vi "calibration sub_VI.vi"(0 "VISA resource ESP32(COM4)":refnum<visa-resource-name>, 1 "Auto \ncalibration \nmode":bool, 2 "OUTPUT_F\nmode":bool, 3 "INPUT_F\nmode":bool, 5 "VISA resource \n2000(COM9)":refnum<visa-resource-name>="COM7", 11 "ESP32 error in":errorcluster, 12 "Calibration \nChannel":string, 13 "Ouput calibration\nparameter":string, 14 "Input calibration\nparameter":string) -> (4 "VISA resource ESP32(COM4) 2":refnum<visa-resource-name>, 6 "Calibration TX":string, 15 "error out":errorcluster)   [LabVIEW 2020]
uses:
  <instrlib>/Keithley 2600 Series/Public/Channel.ctl
  <instrlib>/Keithley 2000/Public/Configure/Configure DC Volts.vi
  <instrlib>/Keithley 2000/Keithley 2000.lvlib
  <instrlib>/Keithley 2600 Series/Keithley 2600 Series.lvlib
panel:
  in  "VISA resource \n2604B(COM10)":refnum<visa-resource-name>="COM7"
  out "OUTPUT or INPUT":u8(slide) scale=0.0..100.0
  out "CALIBRATION":u8(slide) scale=0.0..100.0
  in  "Channel (Channel A)":T1
  out "output parameter":dbl[](array[numeric]) format="%#.2f"
  out "Ouput 2600 read\n(each value)":dbl[][](array[numeric])
  out "Array 3":bool[](array[boolean])
  out "Array 2":i32[](array[numeric])
  in  "Ring":u16(ring)=1 items=["Channel 1"=1, "Channel 2"=2, "Channel 3"=3, "Channel 4"=4]
  # "CHANNEL"
  # "Calibration 吝"
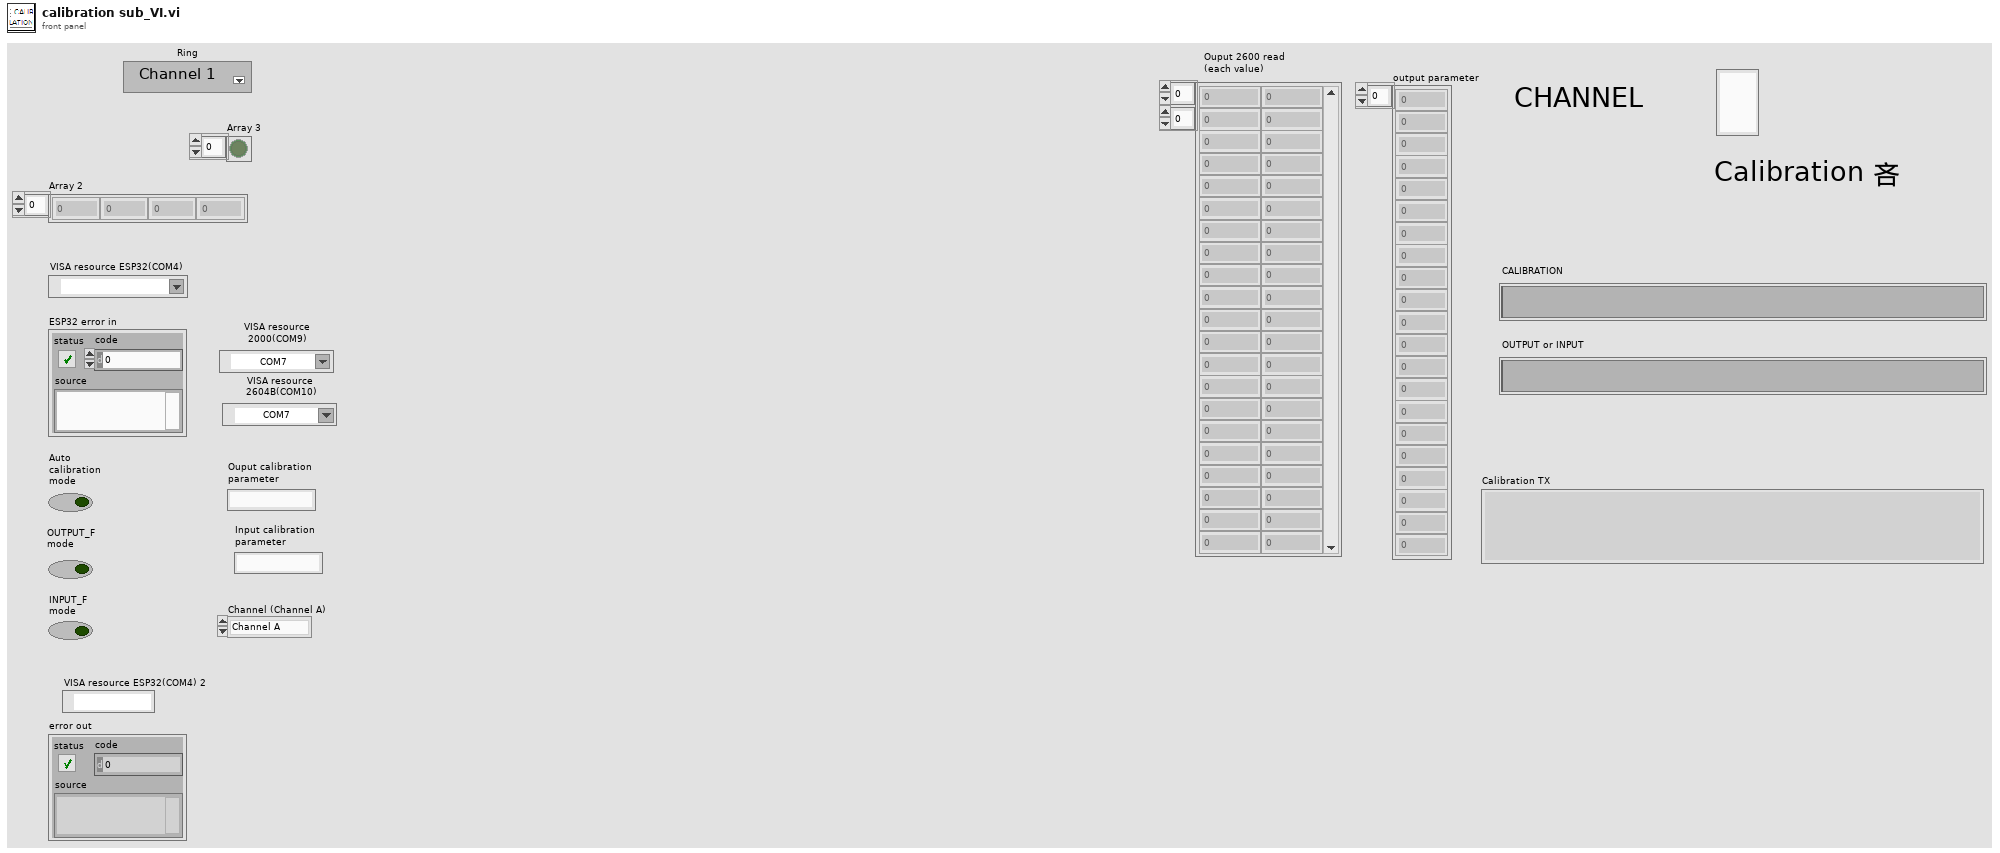
[diagram p1: front panel]
types:
  T1 = typedef "Keithley 2600 Series.lvlib/Channel.ctl" = enum32{"Channel A", "Channel B"}
  T2 = cluster{"Baud Rate":u32, "Parity":u16, "Data Bits":u16, "Stop Bits":u16, "Flow Control":u16}
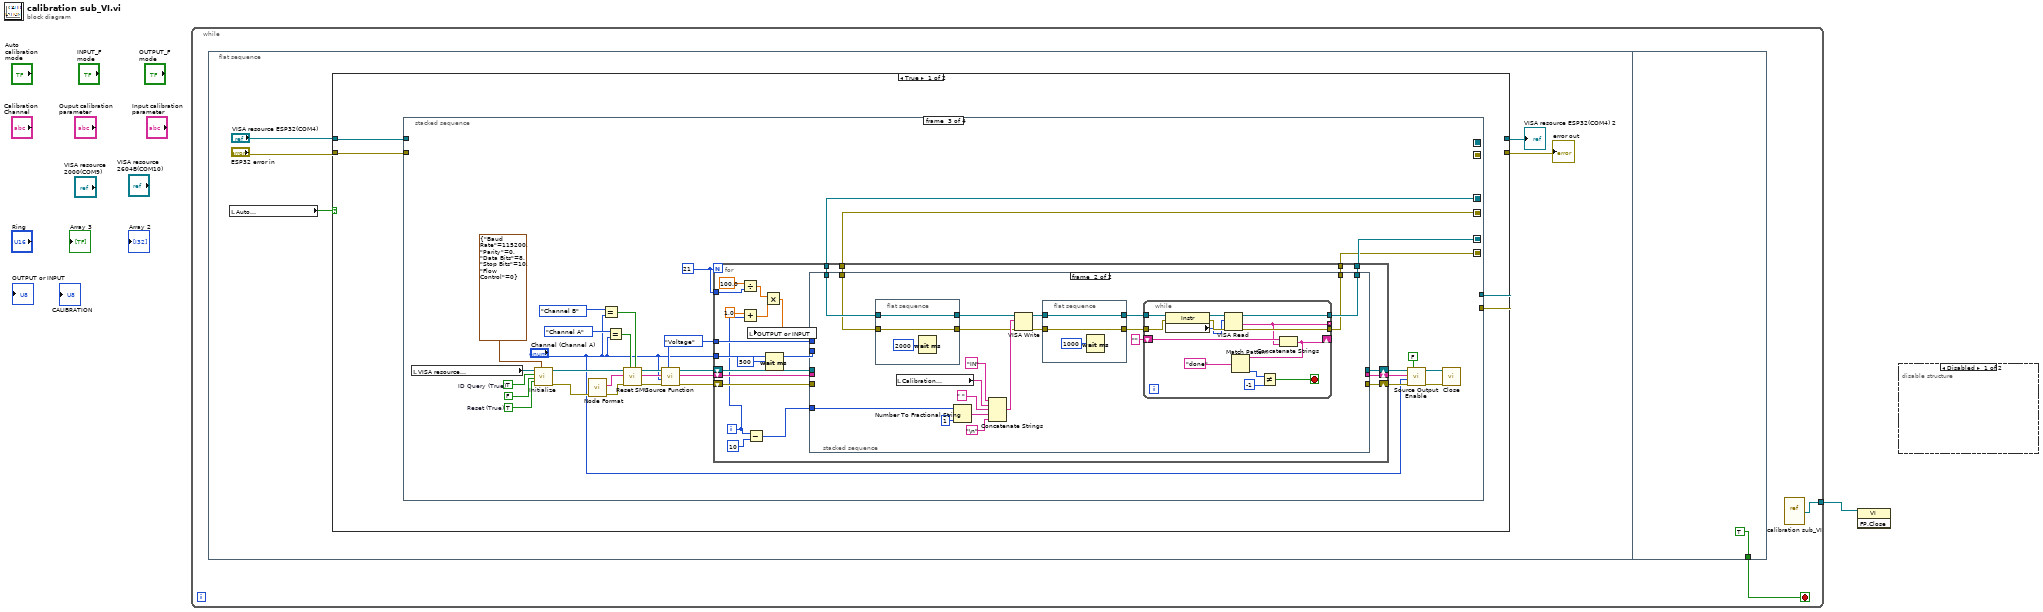
[diagram p0: block diagram]
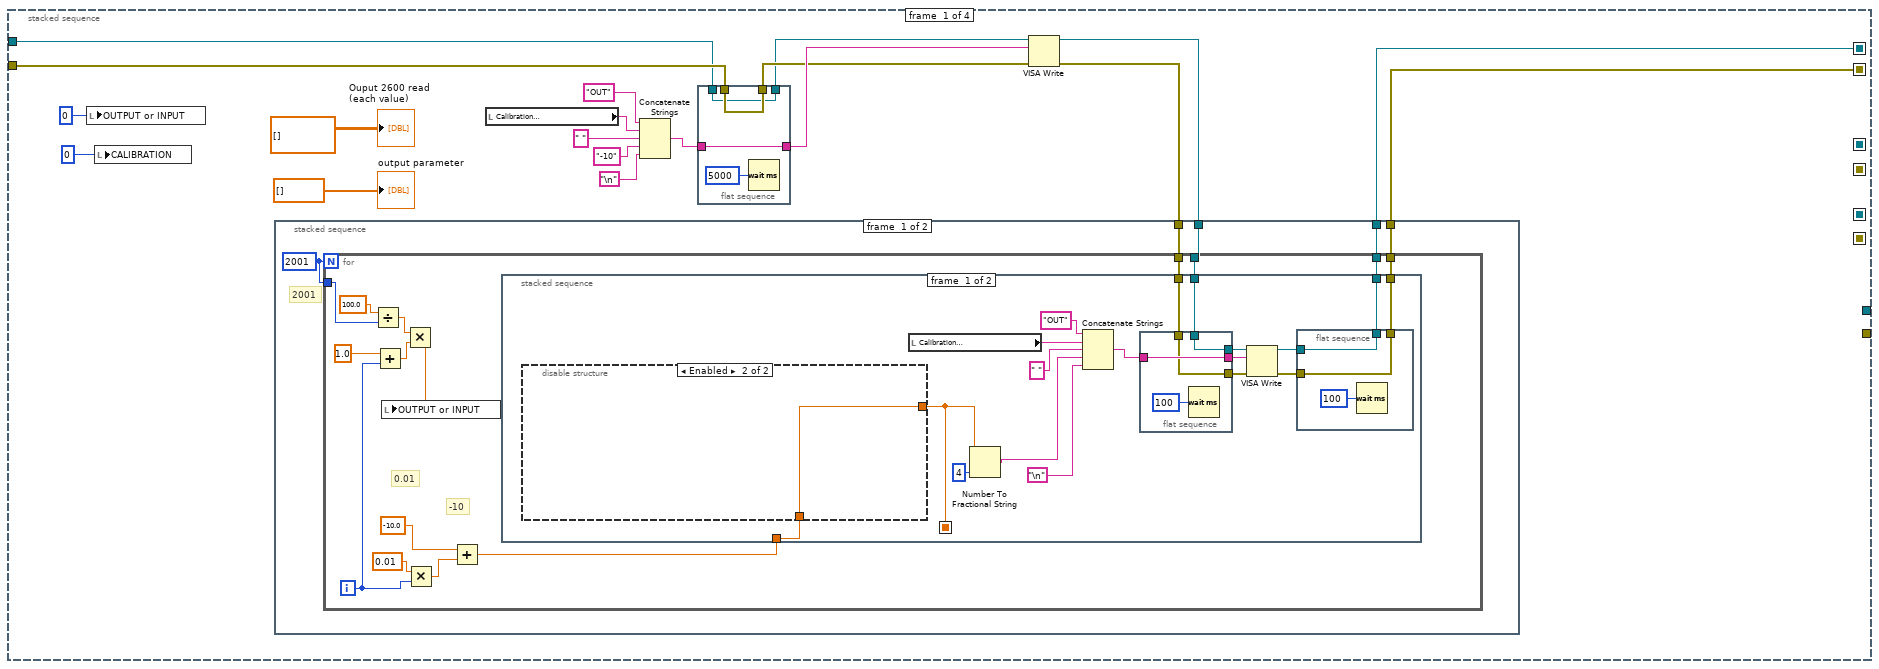
[diagram p3: hidden frame]
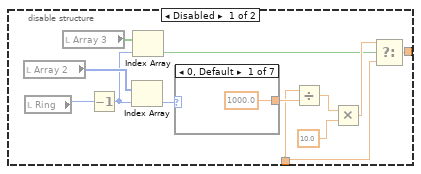
[diagram p4: hidden frame]
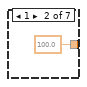
[diagram p5: hidden frame]
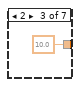
[diagram p6: hidden frame]
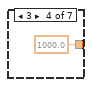
[diagram p7: hidden frame]
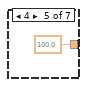
[diagram p8: hidden frame]
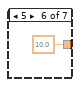
[diagram p9: hidden frame]
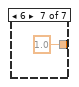
[diagram p10: hidden frame]
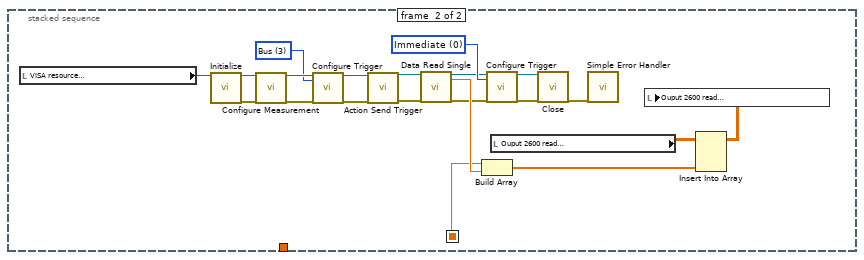
[diagram p11: hidden frame]
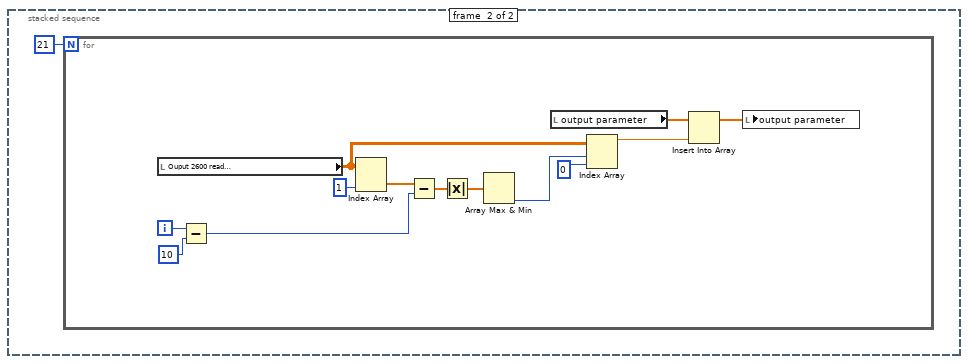
[diagram p12: hidden frame]
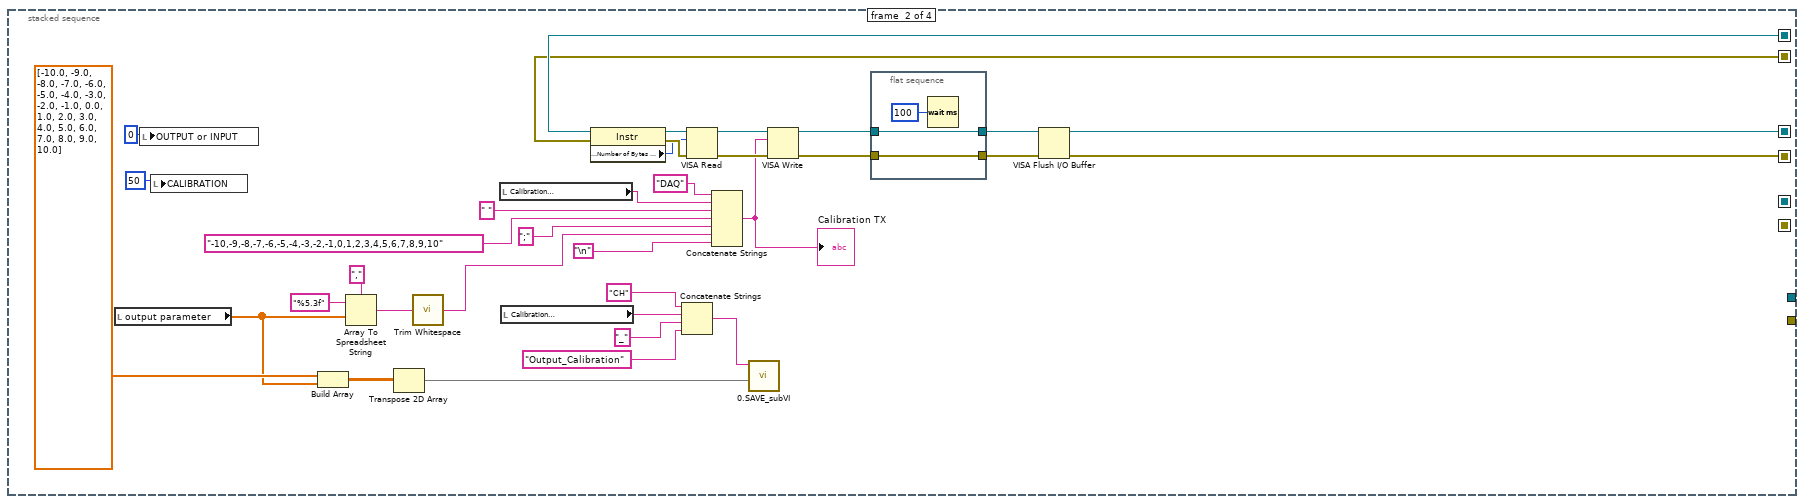
[diagram p13: hidden frame]
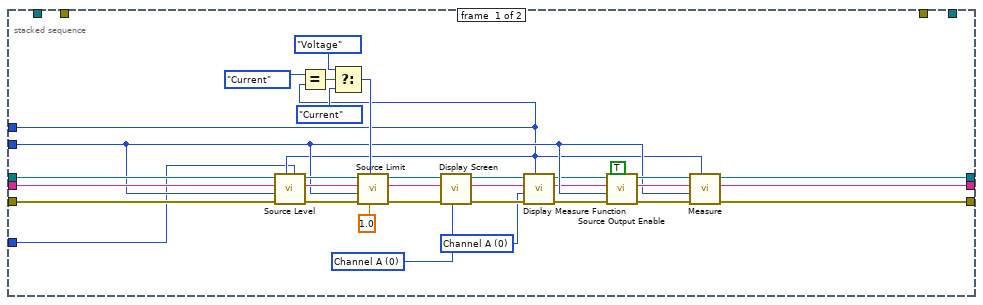
[diagram p14: hidden frame]
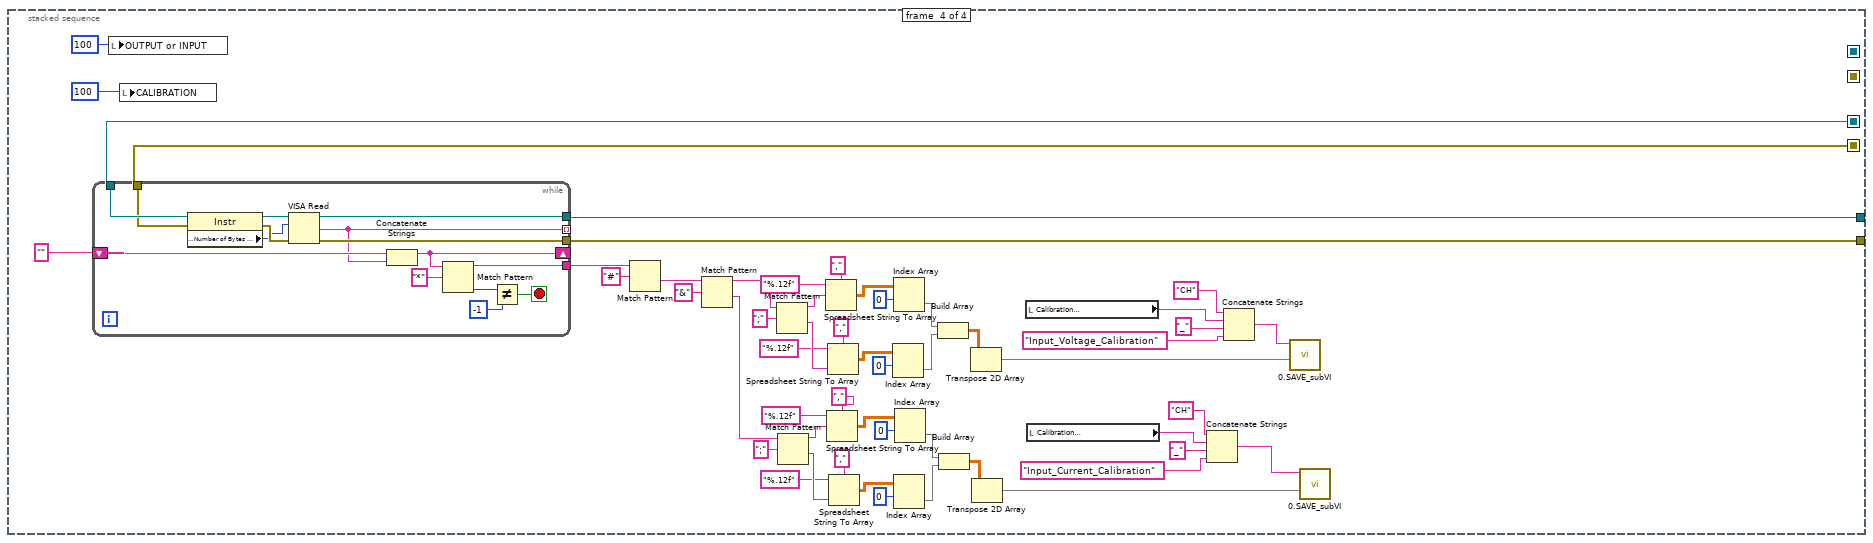
[diagram p15: hidden frame]
diagram:
  n1 = while {
    tunnel: [w2] -> w1
    stop <- w3 stop-if-true
    n2 = flat-sequence {
      tunnel: [TRUE] -> w3
      frame #0 {
        n3 = local read "Auto \ncalibration \nmode"() -> (w4:bool)
        n4 = case shown="True" w4 {
          tunnel: "VISA resource ESP32(COM4)" -> [w12 w369]
          tunnel: [w10 w369] -> w6
          tunnel: [w9 w368] -> w5
          tunnel: "ESP32 error in" -> [w11 w368]
          frame True {
            n5 = stacked-sequence {
              seq-local: [w30 _ _ _] -> [_ w161 _ _]
              seq-local: [w29 _ _ _] -> [_ w160 _ _]
              seq-local: [_ w164 _ _] -> [_ _ w179 _]
              seq-local: [_ w165 _ _] -> [_ _ w180 _]
              seq-local: [_ _ w178 _] -> [_ _ _ w351]
              seq-local: [_ _ w177 _] -> [_ _ _ w350]
              tunnel: w12 -> [w21 _ _ _]
              tunnel: w11 -> [w22 _ _ _]
              tunnel: [_ _ _ w339] -> w10
              tunnel: [_ _ _ w338] -> w9
              frame #0 {
                n6 = local write "OUTPUT or INPUT"(u8 0 ("Slide 2")) -> ()
                n7 = local write "CALIBRATION"(u8 0 ("Slide")) -> ()
                n8 = local read "Calibration \nChannel"() -> (w18:string)
                n9 = Concatenate Strings("OUT" ("string"), w18, " " ("string"), "-10" ("string"), "\n") -> (w25:string)
                n10 = flat-sequence {
                  tunnel: w25 -> [w34]
                  tunnel: [w34] -> w24
                  tunnel: [w33] -> w23
                  tunnel: w22 -> [w33]
                  tunnel: w21 -> [w32]
                  tunnel: [w32] -> w20
                  frame #0 {
                    n11 = Wait (ms)(milliseconds to wait=u32 5000) -> ()  [unwired: 1 out]
                  }
                }
                n12 = VISA Write(VISA resource name=w20, write buffer=w24, error in (no error)=w23) -> (VISA resource name out=w27:refnum<visa-resource-name>, error out=w26:errorcluster)  [unwired: 1 out]
                n13 = stacked-sequence {
                  tunnel: w27 -> [w40 _]
                  tunnel: w26 -> [w39 _]
                  tunnel: [w38 _] -> w30
                  tunnel: [w37 _] -> w29
                  frame #0 {
                    w36 = 2001
                    # "2001"
                    n14 = for {
                      N: w36 -> [_]
                      tunnel: w40 -> [w55]
                      tunnel: w39 -> [w54]
                      tunnel: [w53] -> w38
                      tunnel: [w52] -> w37
                      tunnel: w36 -> [w46]
                      i -> [w44]
                      # "-10"
                      # "0.01"
                      n15 = Divide(x=100.0, y=w46) -> (x/y=w42:dbl)
                      n16 = Add(x=1.0, y=w44) -> (x+y=w43:dbl)
                      n17 = Multiply(x=w42, y=w43) -> (x*y=w41:dbl)
                      n18 = local write "OUTPUT or INPUT"(w41) -> ()
                      n19 = Multiply(x=0.01, y=w44) -> (x*y=w49:dbl)
                      n20 = Add(x=-10.0, y=w49) -> (x+y=w48:dbl)
                      n21 = stacked-sequence {
                        seq-local: [w69 _] -> [_ w107]
                        tunnel: w48 -> [w70 _]
                        tunnel: w55 -> [w65 _]
                        tunnel: w54 -> [w63 _]
                        tunnel: [w62 _] -> w53
                        tunnel: [w60 _] -> w52
                        frame #0 {
                          n22 = disable-structure shown="Enabled" {
                            disable-tunnel: w70 -> [w75 w93]
                            disable-tunnel: [w74 w93] -> w69
                            frame Disabled {
                              n23 = local read "Array 2"() -> (w82:i32[])
                              n24 = local read "Ring"() -> (w83:u16)
                              n25 = local read "Array 3"() -> (w79:bool[])
                              n26 = Decrement(x=w83) -> (x-1=w77:u16)
                              n27 = Index Array(array=w82, index=w77) -> (element=w81:i32)
                              n28 = Index Array(array=w79, index=w77) -> (element=w78:bool)
                              n29 = case shown="0, Default" w81 {
                                tunnel: [1000.0 100.0 10.0 1000.0 100.0 10.0 1.0] -> w84
                                frame 0, Default {
                                }
                                frame 1 {
                                }
                                frame 2 {
                                }
                                frame 3 {
                                }
                                frame 4 {
                                }
                                frame 5 {
                                }
                                frame 6 {
                                }
                              }
                              n30 = Divide(x=w75, y=w84) -> (x/y=w85:dbl)
                              n31 = Multiply(x=w85, y=10.0) -> (x*y=w80:dbl)
                              n32 = Select(t=w80, s=w78, f=w75) -> (s? t:f=w74:dbl)
                            }
                            frame Enabled {
                            }
                          }
                          n33 = local read "Calibration \nChannel"() -> (w57:string)
                          n34 = Number To Fractional String(number=w69, precision (6)=i16 4) -> (F-format string=w73:string)  [unwired: 2 in]
                          n35 = Concatenate Strings("OUT" ("string"), w57, " " ("string"), w73, "\n") -> (w67:string)
                          n36 = flat-sequence {
                            tunnel: [w99] -> w68
                            tunnel: w67 -> [w99]
                            tunnel: [w98] -> w66
                            tunnel: w65 -> [w98]
                            tunnel: [w97] -> w64
                            tunnel: w63 -> [w97]
                            frame #0 {
                              n37 = Wait (ms)(milliseconds to wait=u32 100) -> ()  [unwired: 1 out]
                            }
                          }
                          n38 = VISA Write(VISA resource name=w66, write buffer=w68, error in (no error)=w64) -> (VISA resource name out=w61:refnum<visa-resource-name>, error out=w59:errorcluster)  [unwired: 1 out]
                          n39 = flat-sequence {
                            tunnel: [w95] -> w62
                            tunnel: w61 -> [w95]
                            tunnel: [w94] -> w60
                            tunnel: w59 -> [w94]
                            frame #0 {
                              n40 = Wait (ms)(milliseconds to wait=u32 100) -> ()  [unwired: 1 out]
                            }
                          }
                        }
                        frame #1 {
                          w106 = u16 0 items=["Immediate", "Timer", "Manual", "Bus", "External"] ("Source (0: Immediate)")
                          w116 = u16 3 items=["Immediate", "Timer", "Manual", "Bus", "External"] ("Source (0: Immediate)")
                          n41 = local read "VISA resource \n2000(COM9)"() -> (w101:refnum<visa-resource-name>)
                          n42 = call <instrlib>:"Initialize.vi"("VISA resource name"=w101) -> ("VISA resource name out"=w120:refnum<visa-resource-name>, "error out"=w121:errorcluster)  [unwired: 17 in]
                          n43 = call-poly <instrlib>:"Configure Measurement.vi"("VISA resource name"=w120, "error in (no error)"=w121) -> ("VISA resource name out"=w117:refnum<visa-resource-name>, "error out"=w118:errorcluster)  [unwired: 16 in]
                          n44 = call <instrlib>:"Configure Trigger.vi"("VISA resource name"=w117, "Source (0: Immediate)"=w116, "error in (no error)"=w118) -> ("VISA resource name out"=w115:refnum<visa-resource-name>, "error out"=w114:errorcluster)  [unwired: 15 in]
                          n45 = call <instrlib>:"Action Send Trigger.vi"("VISA resource name"=w115, "error in (no error)"=w114) -> ("VISA resource name out"=w112:refnum<visa-resource-name>, "error out"=w113:errorcluster)  [unwired: 16 in]
                          n46 = call <instrlib>:"Data Read Single.vi"("VISA resource name"=w112, "error in (no error)"=w113) -> ("VISA resource name out"=w102:refnum<visa-resource-name>, "Measurement"=w109:dbl, "error out"=w103:errorcluster)  [unwired: 13 in, 2 out]
                          n47 = Build Array(w107, w109) -> (w108:dbl[])
                          n48 = call <instrlib>:"Configure Trigger.vi"("VISA resource name"=w102, "Source (0: Immediate)"=w106, "error in (no error)"=w103) -> ("VISA resource name out"=w105:refnum<visa-resource-name>, "error out"=w104:errorcluster)  [unwired: 15 in]
                          n49 = local read "Ouput 2600 read\n(each value)"() -> (w110:dbl[][])
                          n50 = call <instrlib>:"Close.vi"("VISA resource name"=w105, "error in (no error)"=w104) -> ("error out"=w119:errorcluster)  [unwired: 17 in]
                          n51 = call <vilib>:"Simple Error Handler.vi"("error in (no error)"=w119) -> ()  [unwired: 4 in, 5 out]
                          n52 = Insert Into Array(array=w110, new element=w108) -> (w111:dbl[][])  [unwired: 2 in]
                          n53 = local write "Ouput 2600 read\n(each value)"(w111) -> ()
                        }
                      }
                    }
                  }
                  frame #1 {
                    n54 = for {
                      N: 21 -> [_]
                      i -> [w135]
                      n55 = local read "Ouput 2600 read\n(each value)"() -> (w123:dbl[][])
                      n56 = Subtract(x=w135, y=10) -> (x-y=w131:i32)
                      n57 = Index Array(array=w123, index (col)=1 ("disabled index (col)")) -> (element=w132:dbl[])  [unwired: 1 in]
                      n58 = Subtract(x=w132, y=w131) -> (x-y=w130:dbl[])
                      n59 = Absolute Value(x=w130) -> (abs(x)=w129:dbl[])
                      n60 = Array Max & Min(array=w129) -> (min index (indices)=w124:i32)  [unwired: 3 out]
                      n61 = local read "output parameter"() -> (w127:dbl[])
                      n62 = Index Array(array=w123, index (row)=w124, index (col)=0 ("disabled index (col)")) -> (element=w126:dbl)
                      n63 = Insert Into Array(array=w127, new element=w126) -> (w128:dbl[])  [unwired: 1 in]
                      n64 = local write "output parameter"(w128) -> ()
                    }
                  }
                }
                "output parameter" <- dbl[] [] ("array")
                "Ouput 2600 read\n(each value)" <- dbl[][] [] ("array")
              }
              frame #1 {
                n65 = local read "output parameter"() -> (w166:dbl[])
                n66 = local write "OUTPUT or INPUT"(u8 0 ("Slide 2")) -> ()
                n67 = local write "CALIBRATION"(u8 50 ("Slide")) -> ()
                n68 = Build Array(dbl[] [-10.0, -9.0, -8.0, -7.0, -6.0, -5.0, -4.0, -3.0, -2.0, -1.0, 0.0, 1.0, 2.0, 3.0, 4.0, 5.0, 6.0, 7.0, 8.0, 9.0, 10.0], w166) -> (w168:dbl[][])
                n69 = Array To Spreadsheet String(delimiter (Tab)=",", array=w166, 3:"%5.3f" ("format string")) -> (spreadsheet string=w163:string)
                n70 = Transpose 2D Array(2D array=w168) -> (transposed array=w151:dbl[][])
                n71 = call <vilib>:"Trim Whitespace.vi"("string"=w163) -> ("trimmed string"=w148:string)  [unwired: 1 in]
                n72 = local read "Calibration \nChannel"() -> (w142:string)
                n73 = local read "Calibration \nChannel"() -> (w139:string)
                n74 = property class="Instr"(reference=w161, error in=w160) -> (reference out=w159:refnum<visa-resource-name>, error out=w158:errorcluster, "Serial Settings:Number of Bytes at Serial Port"=w157:u32)
                n75 = Concatenate Strings("CH" ("time format string (%c)"), w139, "_" ("time format string (%c)"), "Output_Calibration" ("time format string (%c)")) -> (w144:string)
                n76 = VISA Read(VISA resource name=w159, byte count=w157, error in (no error)=w158) -> (VISA resource name out=w156:refnum<visa-resource-name>, error out=w155:errorcluster)  [unwired: 2 out]
                n77 = Concatenate Strings("DAQ" ("string"), w142, " " ("string"), "-10,-9,-8,-7,-6,-5,-4,-3,-2,-1,0,1,2,3,4,5,6,7,8,9,10" ("string"), ";" ("string"), w148, "\n") -> (w146:string)
                "Calibration TX" <- w146
                n78 = call "0.SAVE_subVI.vi"("2D data"=w151, "file name"=w144) -> ()  [unwired: 10 in]
                n79 = VISA Write(VISA resource name=w156, write buffer=w146, error in (no error)=w155) -> (VISA resource name out=w152:refnum<visa-resource-name>, error out=w154:errorcluster)  [unwired: 1 out]
                n80 = flat-sequence {
                  tunnel: [w173] -> w162
                  tunnel: w154 -> [w173]
                  tunnel: [w172] -> w153
                  tunnel: w152 -> [w172]
                  frame #0 {
                    n81 = Wait (ms)(milliseconds to wait=u32 100) -> ()  [unwired: 1 out]
                  }
                }
                n82 = VISA Flush I/O Buffer(VISA resource name=w153, error in (no error)=w162) -> (VISA resource name out=w165:refnum<visa-resource-name>, error out=w164:errorcluster)  [unwired: 1 in]
              }
              frame #2 {
                w175 = 21
                w188 = enum32{"Current", "Voltage"}."Voltage" ("Source Function (Current)")
                w204 = TRUE  # Reset (True)
                w205 = TRUE  # ID Query (True)
                n83 = local read "VISA resource \n2604B(COM10)"() -> (w174:refnum<visa-resource-name>)
                n84 = call <instrlib>:"Initialize.vi"("Reset (True)"=w204, "Serial Configuration"=T2 {"Baud Rate"=115200, "Parity"=0, "Data Bits"=8, "Stop Bits"=10, "Flow Control"=0}, "Error Query (False)"=FALSE, "ID Query (True)"=w205, "VISA resource name"=w174) -> ("error out"=w193:errorcluster, "VISA resource name out"=w202:refnum<visa-resource-name>)  [unwired: 1 in, 4 out]
                n85 = call <instrlib>:"Node Format.vi"("error in"=w193) -> ("error out"=w192:errorcluster, "Formatted Node"=w194:string)  [unwired: 1 in, 8 out]
                n86 = Equal?(x=enum32{"Channel A", "Channel B"}."Channel B", y="Channel (Channel A)") -> (x = y?=w198:bool)
                n87 = Equal?(x=enum32{"Channel A", "Channel B"}."Channel A", y="Channel (Channel A)") -> (x = y?=w199:bool)
                n88 = call <instrlib>:"Reset SMU.vi"("SMU B (No)"=w198, "SMU A (No)"=w199, "error in (no error)"=w192, "Node In"=w194, "VISA resource name"=w202) -> ("error out"=w197:errorcluster, "Node Out"=w195:string, "VISA resource name out"=w196:refnum<visa-resource-name>)  [unwired: 4 out]
                n89 = call <instrlib>:"Source Function.vi"("Function (Current)"=w188, "error in (no error)"=w197, "Channel (Channel A)"="Channel (Channel A)", "Node In"=w195, "VISA resource name"=w196) -> ("error out"=w189:errorcluster, "Node Out"=w191:string, "VISA resource name out"=w190:refnum<visa-resource-name>)  [unwired: 4 out]
                n90 = for {
                  N: w175 -> [_]
                  tunnel: "Channel (Channel A)" -> [w221]
                  tunnel: w188 -> [w220]
                  shift-right: [w222] -> w183
                  shift-left: w191 -> [w227]
                  shift-right: [w224] -> w184
                  shift-left: w190 -> [w226]
                  shift-right: [w223] -> w182
                  shift-left: w189 -> [w225]
                  tunnel: [w217] -> w178
                  tunnel: [w216] -> w177
                  tunnel: w180 -> [w215]
                  tunnel: w179 -> [w214]
                  tunnel: w175 -> [w211]
                  i -> [w209]
                  n91 = Divide(x=100.0, y=w211) -> (x/y=w208:dbl)
                  n92 = Add(x=1.0, y=w209) -> (x+y=w207:dbl)
                  n93 = Subtract(x=w209, y=10) -> (x-y=w219:i32)
                  n94 = Multiply(x=w208, y=w207) -> (x*y=w206:dbl)
                  n95 = local write "OUTPUT or INPUT"(w206) -> ()
                  n96 = Wait (ms)(milliseconds to wait=u32 500) -> ()  [unwired: 1 out]
                  n97 = stacked-sequence {
                    tunnel: w227 -> [w260 _]
                    tunnel: w226 -> [w259 _]
                    tunnel: w225 -> [w258 _]
                    tunnel: [w253 _] -> w224
                    tunnel: [w252 _] -> w223
                    tunnel: [w248 _] -> w222
                    tunnel: w221 -> [w243 _]
                    tunnel: w220 -> [w230 _]
                    tunnel: w219 -> [w229 w276]
                    tunnel: [_ w279] -> w217
                    tunnel: [_ w278] -> w216
                    tunnel: w215 -> [_ w277]
                    tunnel: w214 -> [_ w275]
                    frame #0 {
                      w231 = u16 0 items=["Channel A", "Channel B"] ("Channel (Channel A)")
                      w241 = u16 0 items=["Channel A", "Channel B", "Channels A & B", "User"] ("Screen (Channels A & B)")
                      n98 = call <instrlib>:"Source Level.vi"("Level (0.000)"=w229, "Function (Current)"=w230, "error in (no error)"=w258, "Channel (Channel A)"=w243, "Node In"=w260, "VISA resource name"=w259) -> ("error out"=w257:errorcluster, "Node Out"=w250:string, "VISA resource name out"=w256:refnum<visa-resource-name>)  [unwired: 3 out]
                      n99 = Equal?(x=enum32{"Current", "Voltage"}."Current", y=w230) -> (x = y?=w246:bool)
                      n100 = Select(t=enum32{"Current", "Voltage"}."Voltage" ("x"), s=w246, f=enum32{"Current", "Voltage"}."Current") -> (s? t:f=w244:enum32{"Current", "Voltage"})
                      n101 = call <instrlib>:"Source Limit.vi"("Limit (0.000)"=1.0, "Function (Current)"=w244, "error in (no error)"=w257, "Channel (Channel A)"=w243, "Node In"=w250, "VISA resource name"=w256) -> ("error out"=w238:errorcluster, "Node Out"=w239:string, "VISA resource name out"=w240:refnum<visa-resource-name>)  [unwired: 3 out]
                      n102 = call <instrlib>:"Display Screen.vi"("Screen (Channels A & B)"=w241, "error in (no error)"=w238, "Node In"=w239, "VISA resource name"=w240) -> ("error out"=w235:errorcluster, "Node Out"=w236:string, "VISA resource name out"=w237:refnum<visa-resource-name>)  [unwired: 4 in, 1 out]
                      n103 = call <instrlib>:"Display Measure Function.vi"("Function (Current)"=w230, "error in (no error)"=w235, "Channel (Channel A)"=w231, "Node In"=w236, "VISA resource name"=w237) -> ("error out"=w232:errorcluster, "Node Out"=w233:string, "VISA resource name out"=w234:refnum<visa-resource-name>)  [unwired: 3 in, 1 out]
                      n104 = call <instrlib>:"Source Output Enable.vi"("Output (Off)"=TRUE, "error in (no error)"=w232, "Channel (Channel A)"=w243, "Node In"=w233, "VISA resource name"=w234) -> ("error out"=w255:errorcluster, "Node Out"=w249:string, "VISA resource name out"=w254:refnum<visa-resource-name>)  [unwired: 4 out]
                      n105 = call <instrlib>:"Measure.vi"("Function (Current)"=w230, "error in (no error)"=w255, "Channel (Channel A)"=w243, "Node In"=w249, "VISA resource name"=w254) -> ("error out"=w252:errorcluster, "Node Out"=w248:string, "VISA resource name out"=w253:refnum<visa-resource-name>)  [unwired: 2 in, 2 out]
                    }
                    frame #1 {
                      n106 = flat-sequence {
                        tunnel: [w299] -> w269
                        tunnel: w277 -> [w299]
                        tunnel: w275 -> [w297]
                        tunnel: [w297] -> w267
                        frame #0 {
                          n107 = Wait (ms)(milliseconds to wait=u32 2000) -> ()  [unwired: 1 out]
                        }
                      }
                      n108 = local read "Calibration \nChannel"() -> (w262:string)
                      n109 = Number To Fractional String(number=w276, precision (6)=i16 1) -> (F-format string=w271:string)  [unwired: 2 in]
                      n110 = Concatenate Strings("IN" ("string"), w262, " " ("string"), w271, "\n") -> (w268:string)
                      n111 = VISA Write(VISA resource name=w269, write buffer=w268, error in (no error)=w267) -> (VISA resource name out=w274:refnum<visa-resource-name>, error out=w273:errorcluster)  [unwired: 1 out]
                      n112 = flat-sequence {
                        tunnel: [w282] -> w266
                        tunnel: w274 -> [w282]
                        tunnel: w273 -> [w280]
                        tunnel: [w280] -> w265
                        frame #0 {
                          n113 = Wait (ms)(milliseconds to wait=u32 1000) -> ()  [unwired: 1 out]
                        }
                      }
                      n114 = while {
                        tunnel: [w296] -> w279
                        tunnel: w266 -> [w293]
                        tunnel: w265 -> [w292]
                        tunnel: [w291] -> w278
                        tunnel: [w284] -> _ mode=indexing
                        shift-right: [w283] -> _
                        shift-left: "" -> [w285]
                        stop <- w286 stop-if-true
                        n115 = property class="Instr"(reference=w293, error in=w292) -> (reference out=w295:refnum<visa-resource-name>, error out=w294:errorcluster, "Serial Settings:Number of Bytes at Serial Port"=w290:u32)
                        n116 = VISA Read(VISA resource name=w295, byte count=w290, error in (no error)=w294) -> (VISA resource name out=w296:refnum<visa-resource-name>, read buffer=w284:string, error out=w291:errorcluster)  [unwired: 1 out]
                        n117 = Concatenate Strings(w285, w284) -> (w283:string)
                        n118 = Match Pattern(string=w283, regular expression="done" ("x")) -> (offset past match=w288:i32)  [unwired: 1 in, 3 out]
                        n119 = Not Equal?(x=w288, y=-1) -> (x != y?=w286:bool)
                      }
                    }
                  }
                }
                n120 = call <instrlib>:"Source Output Enable.vi"("Output (Off)"=FALSE, "error in (no error)"=w182, "Channel (Channel A)"="Channel (Channel A)", "Node In"=w183, "VISA resource name"=w184) -> ("error out"=w186:errorcluster, "VISA resource name out"=w187:refnum<visa-resource-name>)  [unwired: 5 out]
                n121 = call <instrlib>:"Close.vi"("error in (no error)"=w186, "VISA resource name"=w187) -> ()  [unwired: 10 out]
              }
              frame #3 {
                n122 = while {
                  tunnel: [w367] -> w339
                  tunnel: [w364] -> w338
                  tunnel: [w358] -> _ mode=indexing
                  shift-right: [w357] -> _
                  shift-left: "" -> [w359]
                  tunnel: w351 -> [w355]
                  tunnel: w350 -> [w354]
                  tunnel: [w353] -> w334
                  stop <- w356 stop-if-true
                  n123 = property class="Instr"(reference=w355, error in=w354) -> (reference out=w366:refnum<visa-resource-name>, error out=w365:errorcluster, "Serial Settings:Number of Bytes at Serial Port"=w363:u32)
                  n124 = VISA Read(VISA resource name=w366, byte count=w363, error in (no error)=w365) -> (VISA resource name out=w367:refnum<visa-resource-name>, read buffer=w358:string, error out=w364:errorcluster)  [unwired: 1 out]
                  n125 = Concatenate Strings(w359, w358) -> (w357:string)
                  n126 = Match Pattern(string=w357, regular expression="*" ("x")) -> (before substring=w353:string, offset past match=w361:i32)  [unwired: 1 in, 2 out]
                  n127 = Not Equal?(x=w361, y=-1) -> (x != y?=w356:bool)
                }
                n128 = local write "OUTPUT or INPUT"(u8 100 ("Slide 2")) -> ()
                n129 = local write "CALIBRATION"(u8 100 ("Slide")) -> ()
                n130 = Match Pattern(string=w334, regular expression="#") -> (after substring=w336:string)  [unwired: 1 in, 3 out]
                n131 = Match Pattern(string=w336, regular expression="&") -> (before substring=w319:string, after substring=w304:string)  [unwired: 1 in, 2 out]
                n132 = Match Pattern(string=w319, regular expression=";") -> (before substring=w322:string, after substring=w325:string)  [unwired: 1 in, 2 out]
                n133 = Match Pattern(string=w304, regular expression=";") -> (before substring=w307:string, after substring=w310:string)  [unwired: 1 in, 2 out]
                n134 = Spreadsheet String To Array(delimiter (Tab)=",", format string="%.12f", spreadsheet string=w322) -> (array=w326:dbl[][])  [unwired: 1 in]
                n135 = Spreadsheet String To Array(delimiter (Tab)=",", format string="%.12f", spreadsheet string=w307) -> (array=w311:dbl[][])  [unwired: 1 in]
                n136 = Spreadsheet String To Array(delimiter (Tab)=",", format string="%.12f", spreadsheet string=w325) -> (array=w331:dbl[][])  [unwired: 1 in]
                n137 = Spreadsheet String To Array(delimiter (Tab)=",", format string="%.12f", spreadsheet string=w310) -> (array=w316:dbl[][])  [unwired: 1 in]
                n138 = Index Array(array=w331, index (row)=0 ("disabled index (col)")) -> (element=w332:dbl[])  [unwired: 1 in]
                n139 = Index Array(array=w326, index (row)=0 ("disabled index (col)")) -> (element=w327:dbl[])  [unwired: 1 in]
                n140 = Index Array(array=w316, index (row)=0 ("disabled index (col)")) -> (element=w317:dbl[])  [unwired: 1 in]
                n141 = Index Array(array=w311, index (row)=0 ("disabled index (col)")) -> (element=w312:dbl[])  [unwired: 1 in]
                n142 = Build Array(w327, w332) -> (w329:dbl[][])
                n143 = Build Array(w312, w317) -> (w314:dbl[][])
                n144 = Transpose 2D Array(2D array=w329) -> (transposed array=w318:dbl[][])
                n145 = Transpose 2D Array(2D array=w314) -> (transposed array=w303:dbl[][])
                n146 = local read "Calibration \nChannel"() -> (w341:string)
                n147 = local read "Calibration \nChannel"() -> (w344:string)
                n148 = Concatenate Strings("CH" ("string"), w344, "_" ("string"), "Input_Current_Calibration" ("time format string (%c)")) -> (w348:string)
                n149 = Concatenate Strings("CH" ("string"), w341, "_" ("string"), "Input_Voltage_Calibration" ("time format string (%c)")) -> (w347:string)
                n150 = call "0.SAVE_subVI.vi"("2D data"=w318, "file name"=w347) -> ()  [unwired: 10 in]
                n151 = call "0.SAVE_subVI.vi"("2D data"=w303, "file name"=w348) -> ()  [unwired: 10 in]
              }
            }
          }
          frame False {
          }
        }
        "VISA resource ESP32(COM4) 2" <- w6
        "error out" <- w5
      }
      frame #1 {
      }
    }
    n152 = vi-ref "calibration sub_VI.vi"() -> (w2:refnum<vi>)
  }
  n153 = invoke class="VI" method="FP.Close"(reference=w1) -> ()  [unwired: 2 in, 3 out]
  n154 = disable-structure shown="Disabled" {
    frame Disabled {
    }
    frame Enabled {
    }
  }
